vi "Get Integer Value.vi"(6 "Default Value":i32, 8 "error in (no error)":errorcluster, 10 "Name":string, 11 "Test Recipe in":refnum<class "Test Recipe.lvclass">) -> (0 "error out":errorcluster, 1 "found?":bool, 2 "Value":i32, 3 "Test Recipe out":refnum<class "Test Recipe.lvclass">)   [LabVIEW 2017, in "Test Recipe.lvlib" / "Test Recipe.lvclass"]
uses:
  Test Recipe.lvclass
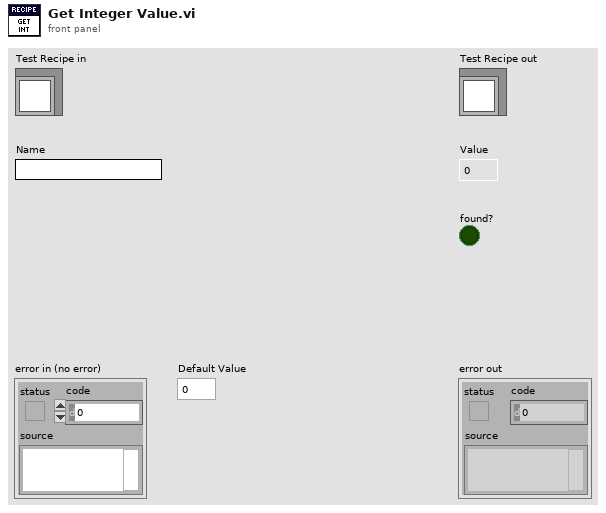
[diagram p1: front panel]
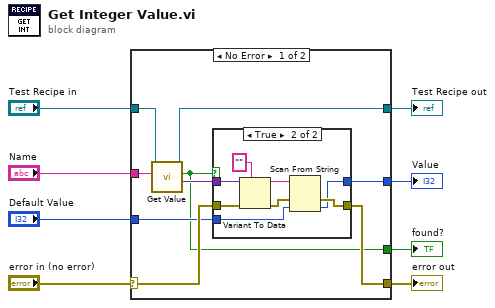
[diagram p0: block diagram]
diagram:
  n1 = case shown="No Error" "error in (no error)" {
    selector: "error in (no error)" -> [w13 w29]
    tunnel: [w10 w29] -> w7
    tunnel: [w16 w28] -> w5
    tunnel: "Test Recipe in" -> [w17 w28]
    tunnel: "Name" -> [w15 _]
    tunnel: [w11 _] -> w3
    tunnel: "Default Value" -> [w12 _]
    tunnel: [w9 _] -> w1
    frame No Error {
      n2 = call-dynamic "Get Value.vi"("Key"=w15, "Registry in"=w17) -> ("Value"=w14:variant, "found?"=w9:bool, "Registry out"=w16:refnum<class "Test Recipe.lvclass">)  [unwired: 6 in, 1 out]
      n3 = case shown="True" w9 {
        tunnel: w14 -> [_ w27]
        tunnel: [w18 w21] -> w11
        tunnel: w13 -> [w19 w26]
        tunnel: [w19 w22] -> w10
        tunnel: w12 -> [w18 w20]
        frame False {
        }
        frame True {
          n4 = Variant To Data(error in=w26, type="", Variant=w27) -> (data=w24:string, error out=w23:errorcluster)
          n5 = Scan From String(input string=w24, error in=w23, default 1=w20) -> (error out=w22:errorcluster, output 1=w21:i32)  [unwired: 2 in, 2 out]
        }
      }
    }
    frame Error {
    }
  }
  "error out" <- w7
  "Test Recipe out" <- w5
  "Value" <- w3
  "found?" <- w1
